vi "runCI1_img.vi"   [LabVIEW 2013]
types:
  T1 = typedef "LVRectTypeDef.ctl" = cluster{"Left":i16, "Top":i16, "Right":i16, "Bottom":i16}
  T2 = cluster{"Xpixels":i32, "Vxminref":dbl, "Vxmaxref":dbl, "P":dbl, "Ypixels":i32, "Vyminref":dbl, "Vymaxref":dbl, "srate":sgl, "sAOxy":i32, "timeout":dbl, "type":string, "date":string, "time":string, "Colormap":u16, "Drawing Mode":u16, "Scanning Mode":u16, "square pixels":bool, "square matrix":bool, "Xpixels Img":i32, "Vx-min Img":dbl, "VX-max Img":dbl, "Ypixels Img":i32, "Vy-min Img":dbl, "Vy-max Img ":dbl, "Angle Img":dbl, "autoshutter":bool, "finite":bool, "cont":bool, "wavdet":bool, "measpoints":i32, "avpp":i32, "bufferAO":i32, "bufferAI":i32, "starttick":u32, "waveform":path, "Vx-ref":dbl, "Vy-ref":dbl, "refreshrate":dbl, "refreshbuffer":i32, "tt_cycles":i32, "motorref":refnum<k7>, "mirrorswitch":refnum<k7>, "sample mode":i32, "maxbufferAI":i32, "sampletreshold":dbl, "srateAODO":sgl, "bin":sgl, "Pel":sgl, "Angle draw":dbl, "srate Img":sgl, "ROIimg_plotbounds":T1, "auto OD":bool, "ODfilt":u16, "reset AO_DO":bool, "aAI":i32[], "aCI":i32[], "aAO":i32[], "aDO":i32[]}
  T3 = cluster{"CI":refnum<k21>[], "E_CI":errorcluster[]}
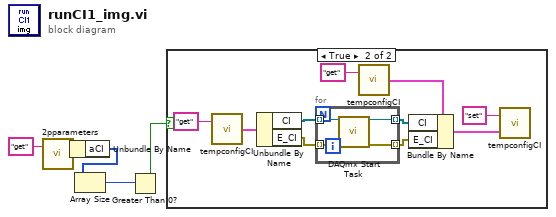
[diagram p0: block diagram]
diagram:
  n1 = call "2pparameters.vi"("command"="get") -> ("params out"=w4:T2)  [unwired: 1 in]
  n2 = Unbundle By Name(w4) -> ("aCI"=w3:i32[])
  n3 = Array Size(array=w3) -> (size(s)=w2:i32)
  n4 = Greater Than 0?(x=w2) -> (x > 0?=w1:bool)
  n5 = case shown="True" w1 {
    frame False {
    }
    frame True {
      n6 = call "tempconfigCI.vi"("command"="get") -> ("Temp Config out"=w13:T3)  [unwired: 1 in]
      n7 = Unbundle By Name(w13) -> ("CI"=w14:refnum<k21>[], "E_CI"=w15:errorcluster[])
      n8 = for {
        tunnel: w15 -> [w19] mode=indexing
        tunnel: w14 -> [w18] mode=indexing
        tunnel: [w17] -> w11 mode=indexing
        tunnel: [w16] -> w10 mode=indexing
        n9 = call <vilib>:"DAQmx Start Task.vi"("task/channels in"=w18, "error in"=w19) -> ("task out"=w17:refnum<k21>, "error out"=w16:errorcluster)  [unwired: 12 in]
      }
      n10 = call "tempconfigCI.vi"("command"="get") -> ("Temp Config out"=w9:T3)  [unwired: 1 in]
      n11 = Bundle By Name(cluster=w9, "CI"=w11, "E_CI"=w10) -> (w6:T3)
      n12 = call "tempconfigCI.vi"("Temp Config in"=w6, "command"="set") -> ()  [unwired: 1 out]
    }
  }
